vi "Servo MSMT GSM Set DC Params.vi"(8 "error in (no error)":errorcluster, 10 "Step In":refnum<k7>, 11 "Servo MSMT in":refnum<class "Servo MSMT.lvclass">) -> (0 "error out":errorcluster, 2 "Step Out":refnum<k7>, 3 "Servo MSMT out":refnum<class "Servo MSMT.lvclass">)   [LabVIEW 2018, in "Servo MSMT.lvlib" / "Servo MSMT.lvclass"]
uses:
  Servo MSMT.lvclass
  C:/Sequence Automation/Plugins/Measurement Interface.lvlibp/Measurement Interface.lvclass
  Servo MSMT.lvclass/Servo MSMT.ctl
  Protected Methods/Read DC Pins.vi
  Protected Methods/Read PAE Pins.vi
  Plugins/Measurement Interface.lvlibp/Private Methods/Engine Reference/Read Engine Reference.vi
  Plugins/TestStand API Tools (TSAT).lvlibp/Step Actions/TSAT Step Actions.lvlib
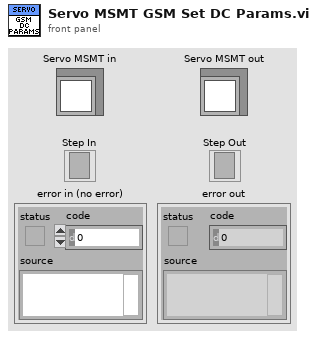
[diagram p1: front panel]
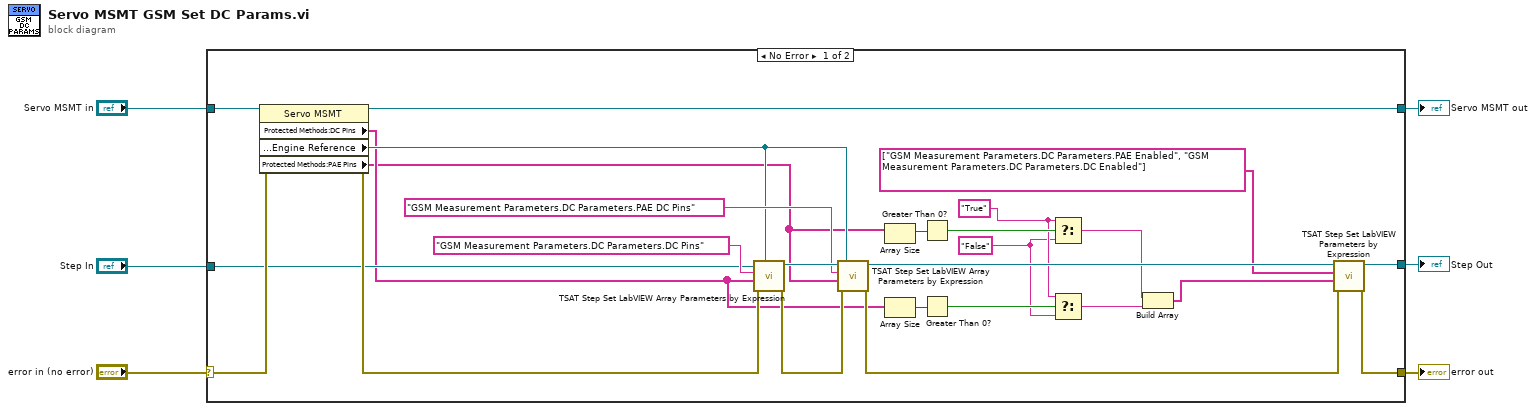
[diagram p0: block diagram]
diagram:
  n1 = case shown="No Error" "error in (no error)" {
    selector: "error in (no error)" -> [w32 w35]
    tunnel: [w19 w35] -> w5
    tunnel: [w30 w34] -> w3
    tunnel: "Servo MSMT in" -> [w31 w34]
    tunnel: "Step In" -> [w25 w33]
    tunnel: [w21 w33] -> w1
    frame No Error {
      w8 = "False"
      w12 = "True"
      n2 = property class="Servo MSMT"(reference=w31, error in=w32) -> (reference out=w30:refnum<class "Servo MSMT.lvclass">, error out=w29:errorcluster, "Protected Methods:DC Pins"=w17:string[], "Protected Methods:Engine Reference"=w23:refnum<k7>, "Protected Methods:PAE Pins"=w7:string[])
      n3 = call "TSAT Step Set LabVIEW Array Parameters by Expression.vi"("Engine In"=w23, "Error In"=w29, "Value Expressions"=w17, "Parameter to Set"="GSM Measurement Parameters.DC Parameters.DC Pins", "Step In"=w25) -> ("Error Out"=w27:errorcluster, "Step Out"=w26:refnum<k7>)  [unwired: 5 in]
      n4 = call "TSAT Step Set LabVIEW Array Parameters by Expression.vi"("Engine In"=w23, "Error In"=w27, "Value Expressions"=w7, "Parameter to Set"="GSM Measurement Parameters.DC Parameters.PAE DC Pins", "Step In"=w26) -> ("Error Out"=w20:errorcluster, "Step Out"=w22:refnum<k7>)  [unwired: 5 in]
      n5 = Array Size(array=w7) -> (size(s)=w16:i32)
      n6 = Array Size(array=w17) -> (size(s)=w13:i32)
      n7 = Greater Than 0?(x=w16) -> (x > 0?=w15:bool)
      n8 = Greater Than 0?(x=w13) -> (x > 0?=w14:bool)
      n9 = Select(t=w12, s=w15, f=w8) -> (s? t:f=w11:string)
      n10 = Select(t=w12, s=w14, f=w8) -> (s? t:f=w10:string)
      n11 = Build Array(w11, w10) -> (w9:string[])
      n12 = call "TSAT Step Set LabVIEW Parameters by Expression.vi"("Error In"=w20, "Value Expressions"=w9, "Parameters to Set"=string[] ["GSM Measurement Parameters.DC Parameters.PAE Enabled", "GSM Measurement Parameters.DC Parameters.DC Enabled"], "Step In"=w22) -> ("Error Out"=w19:errorcluster, "Step Out"=w21:refnum<k7>)  [unwired: 6 in]
    }
    frame Error {
    }
  }
  "error out" <- w5
  "Servo MSMT out" <- w3
  "Step Out" <- w1
